vi "checkCmdIdRule.vi"(8 "error in (no error)":errorcluster, 10 "tcpPacket":T1, 11 "tcpServerCmd in":refnum<class "TcpServerCmd.lvclass">) -> (0 "error out":errorcluster, 1 "ackIterations":i32, 2 "tcpPacket":T1, 3 "tcpServerCmd out":refnum<class "TcpServerCmd.lvclass">)   [LabVIEW 2018, in "TcpServerCmd.lvclass"]
doc: "Get the cmdId sent by TCP Client and compare with lastCmdId saved."
uses:
  TcpServerCmd.lvclass
  home/pcortes/github/ts_labview_tcp_json/src/TcpServerBase/TcpServerBase.lvclass
  TcpServerBase/typedef/tcpPacketTypeDef.ctl
  TcpServerBase/TcpServerBase.lvclass/TcpServerBase.ctl
  TcpServerBase/TcpServerBase.lvclass
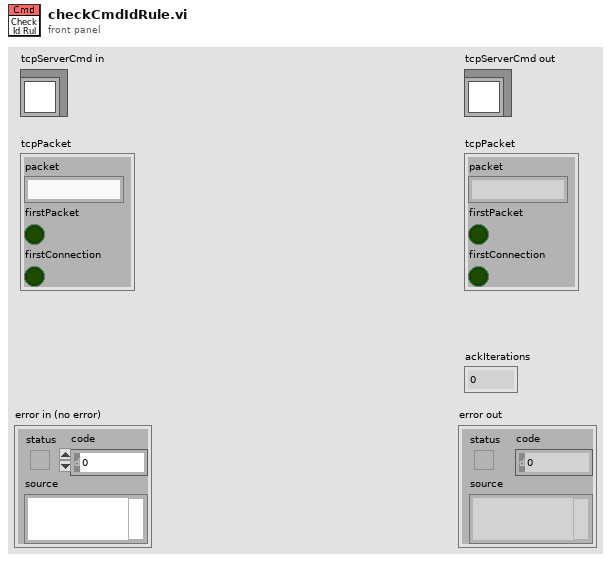
[diagram p1: front panel]
types:
  T1 = typedef "TcpServerBase.lvclass/tcpPacketTypeDef.ctl" = cluster{"packet":string, "firstPacket":bool, "firstConnection":bool}
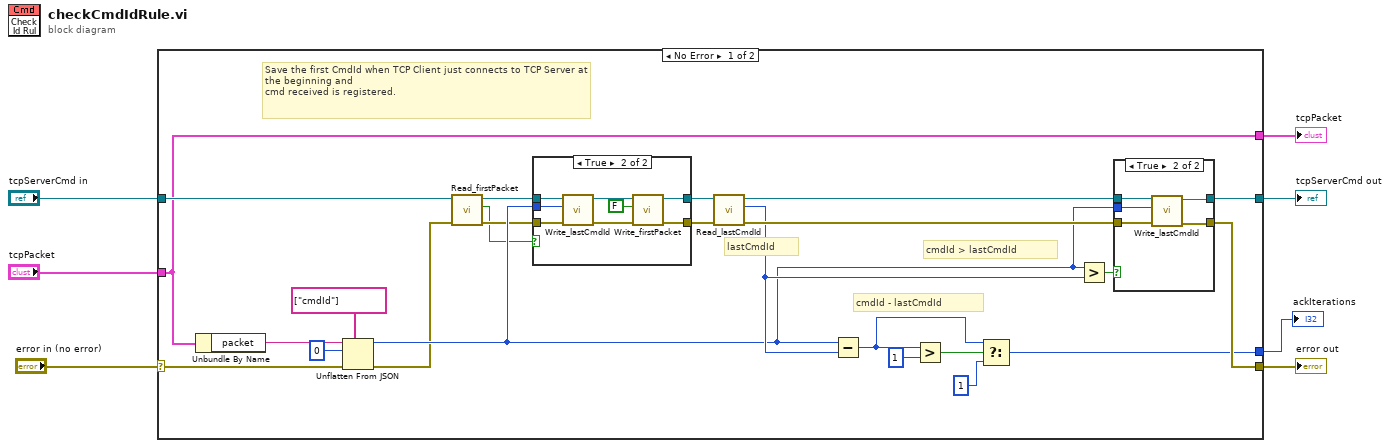
[diagram p0: block diagram]
diagram:
  n1 = case shown="No Error" "error in (no error)" {
    selector: "error in (no error)" -> [w28 w51]
    tunnel: [w25 w51] -> w6
    tunnel: "tcpServerCmd in" -> [w22 w50]
    tunnel: [w27 w50] -> w4
    tunnel: "tcpPacket" -> [w18 w49]
    tunnel: [w18 w49] -> w2
    tunnel: [w12 _] -> w1
    frame No Error {
      # "cmdId > lastCmdId"
      # "cmdId - lastCmdId"
      # "Save the first CmdId when TCP Client just connects to TCP Server at the beginning and\ncmd received is registered."
      # "lastCmdId"
      n2 = Unbundle By Name(w18) -> ("packet"=w29:string)
      n3 = Unflatten From JSON(path=string[] ["cmdId"], JSON string=w29, type and defaults=0, error in (no error)=w28) -> (value=w14:i32, error out=w10:errorcluster)  [unwired: 3 in]
      n4 = call "Read_firstPacket.vi"("error in (no error)"=w10, "TcpServerBase in"=w22) -> ("error out"=w9:errorcluster, "firstPacket"=w8:bool, "TcpServerBase out"=w11:refnum<class "TcpServerCmd.lvclass">)  [unwired: 7 in]
      n5 = case shown="True" w8 {
        tunnel: w11 -> [w33 w41]
        tunnel: w14 -> [_ w38]
        tunnel: [w33 w35] -> w24
        tunnel: [w32 w37] -> w23
        tunnel: w9 -> [w32 w39]
        frame False {
        }
        frame True {
          n6 = call "Write_lastCmdId.vi"("error in (no error)"=w39, "lastCmdId"=w38, "TcpServerBase in"=w41) -> ("error out"=w40:errorcluster, "TcpServerBase out"=w36:refnum<class "TcpServerCmd.lvclass">)  [unwired: 7 in]
          n7 = call "Write_firstPacket.vi"("error in (no error)"=w40, "firstPacket"=FALSE, "TcpServerBase in"=w36) -> ("error out"=w37:errorcluster, "TcpServerBase out"=w35:refnum<class "TcpServerCmd.lvclass">)  [unwired: 7 in]
        }
      }
      n8 = call "Read_lastCmdId.vi"("error in (no error)"=w23, "TcpServerBase in"=w24) -> ("error out"=w26:errorcluster, "lastCmdId"=w15:i32, "TcpServerBase out"=w19:refnum<class "TcpServerCmd.lvclass">)  [unwired: 7 in]
      n9 = Subtract(x=w14, y=w15) -> (x-y=w16:i32)
      n10 = Greater?(x=w16, y=1) -> (0:w20:bool)
      n11 = Select(t=w16, s=w20, f=1) -> (s? t:f=w12:i32)
      n12 = Greater?(x=w14, y=w15) -> (0:w13:bool)
      n13 = case shown="True" w13 {
        tunnel: w19 -> [w43 w48]
        tunnel: [w43 w47] -> w27
        tunnel: w26 -> [w42 w46]
        tunnel: [w42 w45] -> w25
        tunnel: w14 -> [_ w44]
        frame False {
        }
        frame True {
          n14 = call "Write_lastCmdId.vi"("error in (no error)"=w46, "lastCmdId"=w44, "TcpServerBase in"=w48) -> ("error out"=w45:errorcluster, "TcpServerBase out"=w47:refnum<class "TcpServerCmd.lvclass">)  [unwired: 7 in]
        }
      }
    }
    frame Error {
    }
  }
  "error out" <- w6
  "tcpServerCmd out" <- w4
  "tcpPacket" <- w2
  "ackIterations" <- w1
